vi "SMR_LabVIEW_V7.7.vi"() -> ()   [LabVIEW 2025]
uses:
  <vilib>/DAQmx/write.llb/DAQmx Write (Analog DBL 1Chan 1Samp).vi
  <vilib>/DAQmx/read.llb/DAQmx Read (Analog 1D DBL NChan 1Samp).vi
  <vilib>/DAQmx/read.llb/DAQmx Read (Analog 2D DBL NChan NSamp).vi
  <vilib>/Analysis/baseanly.llb/Mean (DBL).vi
  <vilib>/DAQmx/create/channels.llb/DAQmx Create Channel (AI-Temperature-Thermocouple).vi
  <vilib>/DAQmx/create/channels.llb/DAQmx Create Channel (AI-Voltage-Basic).vi
  <vilib>/DAQmx/create/channels.llb/DAQmx Create Channel (AO-Voltage-Basic).vi
  <vilib>/DAQmx/miscellaneous.llb/DAQmx Fill In Error Info.vi
  <vilib>/DAQmx/configure/timing.llb/DAQmx Timing (Sample Clock).vi
  <vilib>/addons/control/pid/pid.llb/PID (DBL).vi
  <vilib>/measure/maspectr.llb/FFT Power Spectrum and PSD for 1 Chan.vi
  <vilib>/measure/matone.llb/Extract Single Tone Information 1 Chan.vi
  <vilib>/addons/control/pid/NI_PID_pid.lvlib
  <vilib>/Analysis/NI_AALBase.lvlib
  <vilib>/ptbypt/NI_PtbyPt.lvlib
  <vilib>/measure/NI_MAPro.lvlib
panel:
  out "Main Loop Flow (GPM)":dbl
  out "FM Amplitude":dbl
  out "FM Frequency":dbl
  out "Spectrum":cluster{"f0":dbl, "df":dbl, "magnitude":dbl[]}(graph)
  out "Raw Signal":waveform(dbl)(graph)
  out "Smoothed HX Flow (GPM)":dbl
  out "Flow History":dbl(graph)
  out "HX Flow (GPM)":dbl
  out "Voltage Across Rod (V)":dbl format="%0.2f"
  out "Current Run Folder":path
  in  "Log Root Folder":path=path "C:/Users/LocalUser/Documents/GitHub/thermal-loop/resources/v0.1.1/data/001"
  out "Raw NI9201 \nVoltage Display":T1
  in  "Loop Period (ms)":dbl=1000.0
  in  "Stop":bool
  out "Auto Steady State Threshold (deg C/min)":dbl
  out "Max dT/dt (deg C/min)":dbl
  out "Temp Change Rate (deg C/min)":dbl
  out "5-Min Baseline Complete":bool
  out "Rate Window Ready":bool
  out "Steady State":bool
  in  "Voltage Limit (V)":dbl=10.0
  in  "Temperature Limit (C)":dbl=50.0
  in  "Pressure Limit (psi)":dbl=15.0
  out "Max Voltage":bool
  out "Max Temperature":bool
  out "Max Pressure":bool
  out "Heat Exchanger Pressure History":dbl(graph)
  out "Main Loop Pressure History":T2(graph)
  out "Overall Avg Pressure (psi)":dbl
  out "Heat Exchanger Pressure P6 (psi)":dbl
  out "Main Loop Avg Pressure (psi)":dbl
  out "Pressure Display":T3
  out "Overall Pressure History":T4(graph)
  out "Max Loop Pressure (psi)":dbl
  out "Heat Exchanger Temperature History":cluster{"Waveform":dbl, "Waveform":dbl}(graph)
  out "Main Loop Temeperature History":T5(graph)
  out "Heat Exchanger Avg Temp (deg C)":dbl
  out "Temperature Display":T6
  out "Overall Temperature History":T7(graph)
  out "Overall Avg Temp (deg C)":dbl
  out "Max Loop Temp (deg C)":dbl
  out "Final P-Valve Voltage (V)":dbl
  out "PID Trim Voltage (V)":dbl
  in  "PID Temp Setpoint (deg C)":dbl
  in  "Auto PID Enable":bool
  in  "Manual P-Valve Voltage (V)":dbl min=0.0 max=10.0
  out "Main Loop Avg Temp (deg C)":dbl
  # "Heat Exchanger Flow"
  # "Control/Troubleshoot"
  # "Steady State"
  # "Emergency Indicators"
  # "Pressure"
  # "Temperature"
  # "Proportional Valve Control"
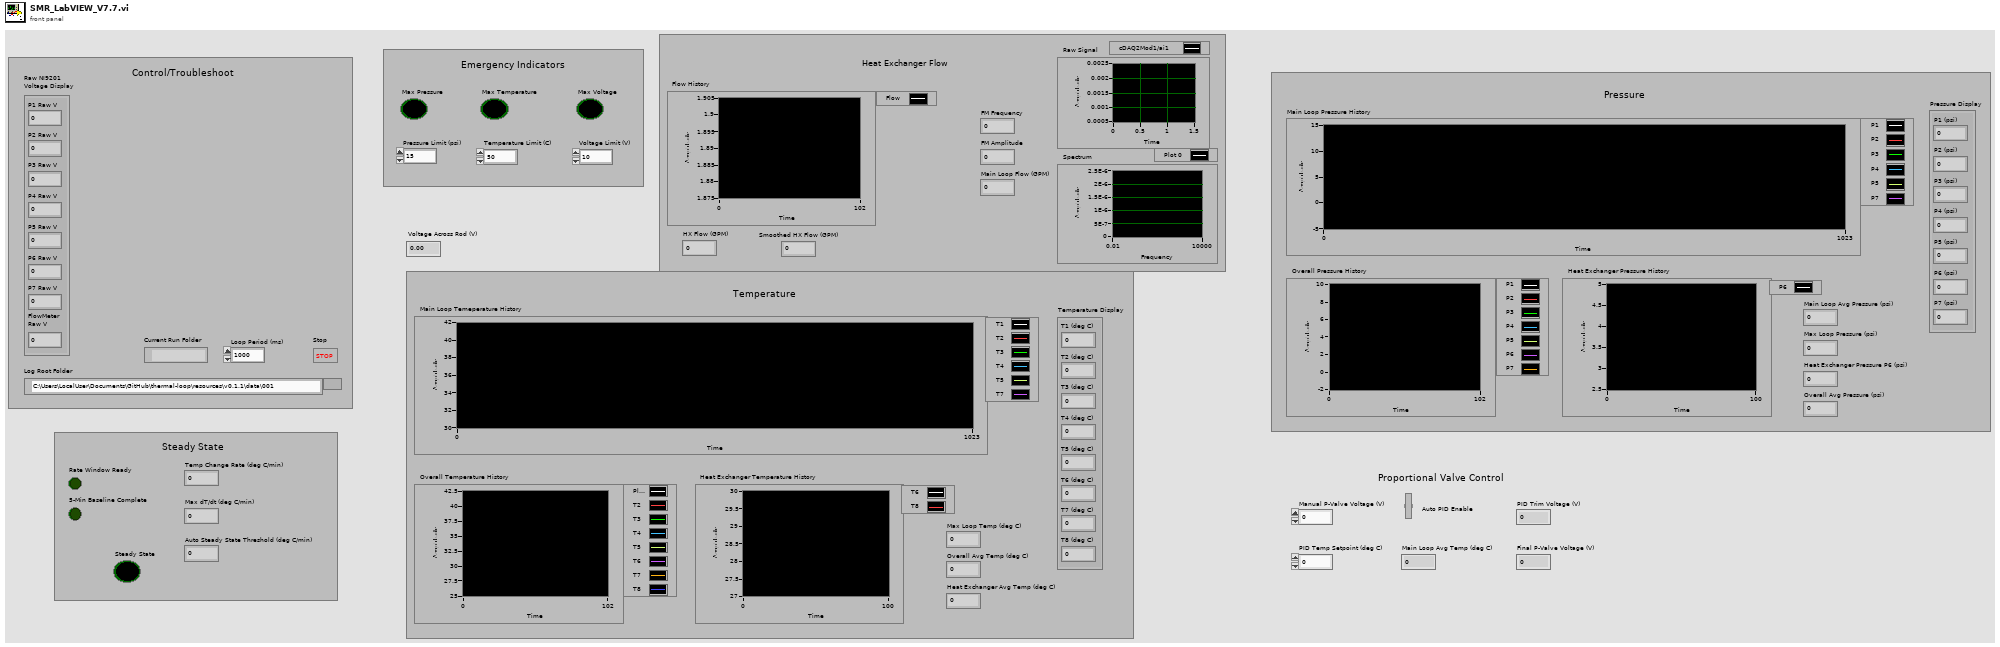
[diagram p1: front panel]
types:
  T1 = cluster{"P1 Raw V":dbl, "P2 Raw V":dbl, "P3 Raw V":dbl, "P4 Raw V":dbl, "P5 Raw V":dbl, "P6 Raw V":dbl, "P7 Raw V":dbl, "FlowMeter\nRaw V":dbl}
  T2 = cluster{"P1":dbl, "P2":dbl, "P3":dbl, "P4":dbl, "P5":dbl, "P7":dbl}
  T3 = cluster{"P1 (psi)":dbl, "P2 (psi)":dbl, "P3 (psi)":dbl, "P4 (psi)":dbl, "P5 (psi)":dbl, "P6 (psi)":dbl, "P7 (psi)":dbl}
  T4 = cluster{"P1":dbl, "P2":dbl, "P3":dbl, "P4":dbl, "P5":dbl, "P6":dbl, "P7":dbl}
  T5 = cluster{"Waveform":dbl, "Waveform":dbl, "Waveform":dbl, "Waveform":dbl, "Waveform":dbl, "Waveform":dbl}
  T6 = cluster{"T1 (deg C)":dbl, "T2 (deg C)":dbl, "T3 (deg C)":dbl, "T4 (deg C)":dbl, "T5 (deg C)":dbl, "T6 (deg C)":dbl, "T7 (deg C)":dbl, "T8 (deg C)":dbl}
  T7 = cluster{"Waveform":dbl, "Waveform":dbl, "Waveform":dbl, "Waveform":dbl, "Waveform":dbl, "Waveform":dbl, "Waveform":dbl, "Waveform":dbl}
  T8 = enum16{"open", "replace", "create", "open or create", "replace or create", "replace or create with confirmation"}
  T9 = cluster{"proportional gain (Kc)":dbl, "integral time (Ti, min)":dbl, "derivative time (Td, min)":dbl}
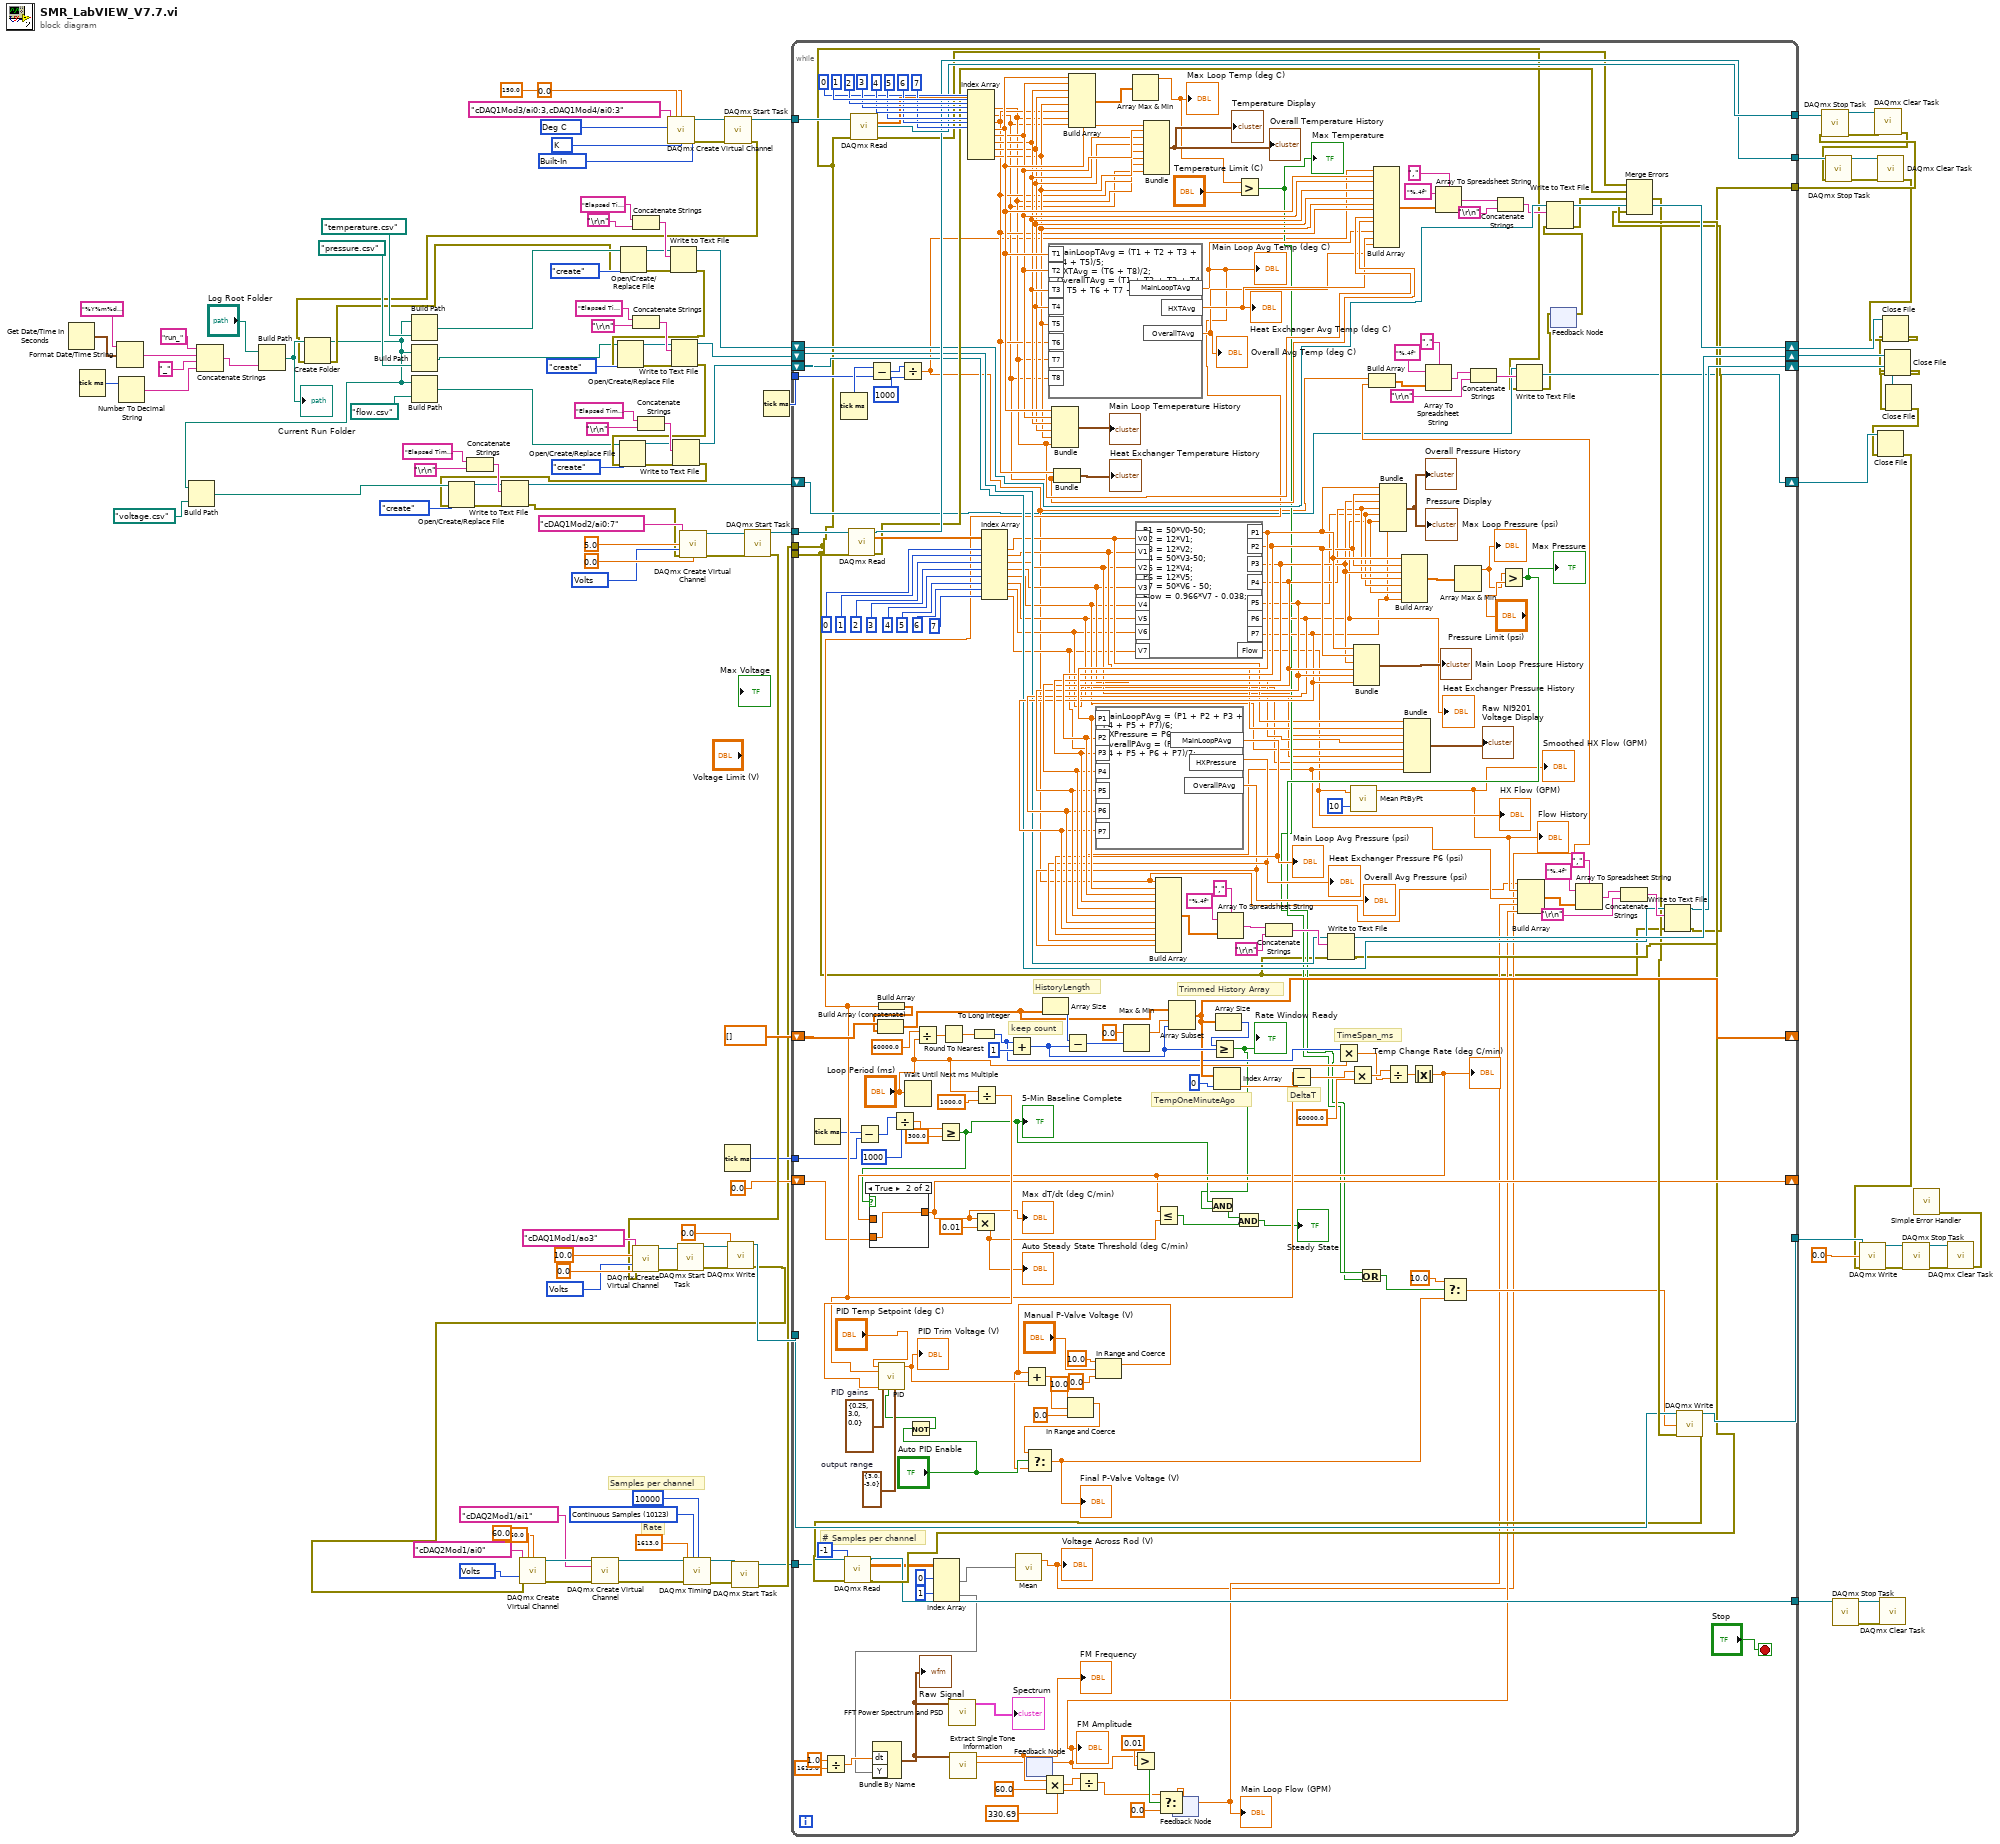
[diagram p0: block diagram]
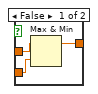
[diagram p2: hidden frame]
diagram:
  w30 = 10123 items=["Finite Samples"=10178, "Continuous Samples"=10123, "Hardware Timed Single Point"=12522] ("sample mode")
  w32 = 10348 items=["Volts"=10348, "From Custom Scale"=10065] ("units")
  w52 = 10348 items=["Volts"=10348, "From Custom Scale"=10065] ("units")
  w116 = 10200 items=["Built-In"=10200, "Constant Value"=10116, "Channel"=10113] ("cjc source")
  w117 = 10073 items=["J"=10072, "K"=10073, "N"=10077, "R"=10082, "S"=10085, "T"=10086, "B"=10047, "E"=10055] ("thermocouple type")
  w118 = 10143 items=["Deg C"=10143, "Deg F"=10144, "Kelvins"=10325, "Deg R"=10145, "From Custom Scale"=10065] ("units")
  w125 = 10348 items=["Volts"=10348, "From Custom Scale"=10065] ("units")
  # "Samples per channel"
  # "Rate"
  n1 = Get Date/Time In Seconds() -> (seconds since 1Jan1904=w74:timestamp)
  n2 = Tick Count (ms)() -> (millisecond timer value=w72:u32)
  n3 = Format Date/Time String(time format string (%c)="%Y%m%d_%H%M%S", seconds (now)=w74) -> (date/time string=w69:string)  [unwired: 1 in]
  n4 = Number To Decimal String(number=w72) -> (decimal integer string=w70:string)  [unwired: 1 in]
  n5 = Concatenate Strings("run_" ("string"), w69, "_" ("string"), w70) -> (w66:string)
  n6 = Build Path(base path="Log Root Folder", name or relative path=w66) -> (appended path=w65:path)
  "Current Run Folder" <- w65
  n7 = Concatenate Strings("Elapsed Time (s), Rod voltage (V)", "\r\n") -> (w14:string)
  n8 = Concatenate Strings("Elapsed Time (s),T1 (deg C),T2 (deg C),T3 (deg C),T4 (deg C),T5 (deg C),T6 (deg C),T7 (deg C),T8 (deg C),Main Loop Avg Temp (deg C),HX Avg Temp (deg C),Overall Avg Temp (deg C)", "\r\n") -> (w99:string)
  n9 = Concatenate Strings("Elapsed Time (s),P1 (psi),P2 (psi),P3 (psi),P4 (psi),P5 (psi),P6 (psi),P7 (psi),Main Loop Avg Pressure (psi),HX Pressure (psi),Overall Avg Pressure (psi)", "\r\n") -> (w97:string)
  n10 = Concatenate Strings("Elapsed Time (s),Heat Exchanger Flow (GPM),Flow Raw Voltage (V), Main Loop Flow (GPM), Flow Signal Amplitude (V)", "\r\n") -> (w93:string)
  n11 = call-poly <vilib>:"DAQmx Create Virtual Channel.vi"("maximum value"=150.0, "minimum value"=0.0, "physical channels"=tag "cDAQ1Mod3/ai0:3,cDAQ1Mod4/ai0:3", "cjc source"=w116, "units"=w118, "thermocouple type"=w117) -> ("task out"=w115:refnum<k21>, "error out"=w114:errorcluster)  [unwired: 8 in]
  n12 = Tick Count (ms)() -> (millisecond timer value=w37:u32)
  n13 = call <vilib>:"DAQmx Start Task.vi"("task/channels in"=w115, "error in"=w114) -> ("task out"=w113:refnum<k21>, "error out"=w58:errorcluster)  [unwired: 12 in]
  n14 = Create Folder(path (use dialog)=w65, error in=w58) -> (created path=w8:path, error out=w57:errorcluster)  [unwired: 1 in, 1 out]
  n15 = Build Path(base path=w8, name or relative path=path "voltage.csv") -> (appended path=w9:path)
  n16 = Build Path(base path=w8, name or relative path=path "temperature.csv") -> (appended path=w64:path)
  n17 = Build Path(base path=w8, name or relative path=path "pressure.csv") -> (appended path=w63:path)
  n18 = Build Path(base path=w8, name or relative path=path "flow.csv") -> (appended path=w62:path)
  n19 = Open/Create/Replace File(file path (use dialog)=w64, error in=w57, operation (0:open)=T8."create") -> (refnum out=w98:refnum<file>, error out=w82:errorcluster)  [unwired: 3 in, 1 out]
  n20 = Write to Text File(file (use dialog)=w98, text=w99, error in=w82) -> (refnum out=w89:refnum<file>, error out=w81:errorcluster)  [unwired: 1 in, 1 out]
  n21 = Open/Create/Replace File(file path (use dialog)=w63, error in=w81, operation (0:open)=T8."create") -> (refnum out=w96:refnum<file>, error out=w80:errorcluster)  [unwired: 3 in, 1 out]
  n22 = Write to Text File(file (use dialog)=w96, text=w97, error in=w80) -> (refnum out=w88:refnum<file>, error out=w79:errorcluster)  [unwired: 1 in, 1 out]
  n23 = Open/Create/Replace File(file path (use dialog)=w62, error in=w79, operation (0:open)=T8."create") -> (refnum out=w92:refnum<file>, error out=w78:errorcluster)  [unwired: 3 in, 1 out]
  n24 = Write to Text File(file (use dialog)=w92, text=w93, error in=w78) -> (refnum out=w87:refnum<file>, error out=w6:errorcluster)  [unwired: 1 in, 1 out]
  n25 = Open/Create/Replace File(file path (use dialog)=w9, error in=w6, operation (0:open)=T8."create") -> (refnum out=w13:refnum<file>, error out=w10:errorcluster)  [unwired: 3 in, 1 out]
  n26 = Write to Text File(file (use dialog)=w13, text=w14, error in=w10) -> (refnum out=w4:refnum<file>, error out=w5:errorcluster)  [unwired: 1 in, 1 out]
  n27 = call-poly <vilib>:"DAQmx Create Virtual Channel.vi"("maximum value"=5.0, "minimum value"=0.0, "physical channels"=tag "cDAQ1Mod2/ai0:7", "units"=w125, "error in"=w5) -> ("task out"=w124:refnum<k21>, "error out"=w123:errorcluster)  [unwired: 9 in]
  n28 = call <vilib>:"DAQmx Start Task.vi"("task/channels in"=w124, "error in"=w123) -> ("task out"=w122:refnum<k21>, "error out"=w45:errorcluster)  [unwired: 12 in]
  n29 = call-poly <vilib>:"DAQmx Create Virtual Channel.vi"("maximum value"=10.0, "minimum value"=0.0, "physical channels"=tag "cDAQ1Mod1/ao3", "units"=w52, "error in"=w45) -> ("task out"=w51:refnum<k21>, "error out"=w50:errorcluster)  [unwired: 9 in]
  n30 = call <vilib>:"DAQmx Start Task.vi"("task/channels in"=w51, "error in"=w50) -> ("task out"=w49:refnum<k21>, "error out"=w48:errorcluster)  [unwired: 12 in]
  n31 = call-poly <vilib>:"DAQmx Write.vi"("task/channels in"=w49, "data"=0.0, "error in"=w48) -> ("task out"=w46:refnum<k21>, "error out"=w24:errorcluster)  [unwired: 10 in, 1 out]
  n32 = call-poly <vilib>:"DAQmx Create Virtual Channel.vi"("maximum value"=60.0, "minimum value"=-60.0, "physical channels"=tag "cDAQ2Mod1/ai0", "units"=w32, "error in"=w24) -> ("task out"=w20:refnum<k21>, "error out"=w19:errorcluster)  [unwired: 9 in]
  n33 = call-poly <vilib>:"DAQmx Create Virtual Channel.vi"("task in"=w20, "physical channels"=tag "cDAQ2Mod1/ai1", "error in"=w19) -> ("task out"=w18:refnum<k21>, "error out"=w17:errorcluster)  [unwired: 11 in]
  n34 = call-poly <vilib>:"DAQmx Timing.vi"("task/channels in"=w18, "sample mode"=w30, "samples per channel"=10000, "rate"=1613.0, "error in"=w17) -> ("task out"=w28:refnum<k21>, "error out"=w27:errorcluster)  [unwired: 9 in]
  n35 = call <vilib>:"DAQmx Start Task.vi"("task/channels in"=w28, "error in"=w27) -> ("task out"=w22:refnum<k21>, "error out"=w23:errorcluster)  [unwired: 12 in]
  n36 = Tick Count (ms)() -> (millisecond timer value=w86:u32)
  n37 = while {
    tunnel: w122 -> [w330]
    tunnel: w113 -> [w313]
    tunnel: [w303] -> w112
    tunnel: [w131] -> _
    tunnel: [w302] -> w111
    tunnel: [w177] -> w110
    shift-right: [w279] -> w85
    shift-left: w89 -> [w280]
    shift-right: [w260] -> w84
    shift-left: w88 -> [w261]
    shift-right: [w252] -> w83
    shift-left: w87 -> [w253]
    tunnel: w86 -> [w298]
    shift-right: [w231] -> _
    shift-left: dbl[] [] -> [w244]
    tunnel: w46 -> [w212]
    tunnel: w23 -> [w131]
    tunnel: [w219] -> w43
    tunnel: w37 -> [w201]
    shift-right: [w194] -> _
    shift-left: 0.0 -> [w196]
    tunnel: w22 -> [w176]
    tunnel: [w175] -> w21
    shift-right: [w132] -> w3
    shift-left: w4 -> [w133]
    stop <- "Stop" stop-if-true
    w217 = cluster{"output high":dbl, "output low":dbl} {"output high"=3.0, "output low"=-3.0}  # output range
    w218 = T9 {"proportional gain (Kc)"=0.25, "integral time (Ti, min)"=3.0, "derivative time (Td, min)"=0.0}  # PID gains
    # "# Samples per channel"
    # "TimeSpan_ms"
    # "DeltaT"
    # "TempOneMinuteAgo"
    # "Trimmed History Array"
    # "HistoryLength"
    # "keep count"
    n38 = Tick Count (ms)() -> (millisecond timer value=w202:u32)
    n39 = Divide(x=1.0, y=1613.0) -> (x/y=w148:dbl)
    n40 = Tick Count (ms)() -> (millisecond timer value=w299:u32)
    n41 = call-poly <vilib>:"DAQmx Read.vi"("task/channels in"=w330, "error in"=w131) -> ("task out"=w302:refnum<k21>, "data"=w321:dbl[], "error out"=w300:errorcluster)  [unwired: 11 in]
    n42 = call-poly <vilib>:"DAQmx Read.vi"("task/channels in"=w313, "error in"=w131) -> ("task out"=w303:refnum<k21>, "data"=w304:dbl[], "error out"=w301:errorcluster)  [unwired: 11 in]
    n43 = Subtract(x=w202, y=w201) -> (x-y=w200:u32)
    n44 = Subtract(x=w299, y=w298) -> (x-y=w297:u32)
    n45 = Divide(x=w200, y=u32 1000) -> (x/y=w198:dbl)
    n46 = Divide(x=w297, y=u32 1000) -> (x/y=w136:dbl)
    n47 = Wait Until Next ms Multiple(millisecond multiple="Loop Period (ms)") -> ()  [unwired: 1 out]
    n48 = Not(x="Auto PID Enable") -> (.not. x?=w213:bool)
    n49 = Divide(x=60000.0, y="Loop Period (ms)") -> (x/y=w241:dbl)
    n50 = Greater Or Equal?(x=w198, y=300.0) -> (x >= y?=w191:bool)
    "5-Min Baseline Complete" <- w191
    n51 = Round To Nearest(number=w241) -> (nearest integer value=w240:dbl)
    n52 = Index Array(array=w304, index #1=0 ("index"), index #2=1 ("index"), index #3=2 ("index"), index #4=3 ("index"), index #5=4 ("index"), index #6=5 ("index"), index #7=6 ("index"), index #8=7 ("index")) -> (element #1=w289:dbl, element #2=w288:dbl, element #3=w290:dbl, element #4=w295:dbl, element #5=w294:dbl, element #6=w293:dbl, element #7=w292:dbl, element #8=w291:dbl)
    n53 = To Long Integer(number=w240) -> (32bit integer=w228:i32)
    n54 = Divide(x="Loop Period (ms)", y=1000.0) -> (x/y=w214:dbl)
    n55 = Index Array(array=w321, index #1=0 ("index"), index #2=1 ("index"), index #3=2 ("index"), index #4=3 ("index"), index #5=4 ("index"), index #6=5 ("index"), index #7=6 ("index"), index #8=7 ("index")) -> (element #1=w174:dbl, element #2=w173:dbl, element #3=w172:dbl, element #4=w171:dbl, element #5=w170:dbl, element #6=w169:dbl, element #7=w168:dbl, element #8=w167:dbl)
    n56 = Add(x=w228, y=1) -> (x+y=w233:i32)
    n57 = feedback #1() -> (w144:dbl)  [unwired: 1 in]
    "FM Amplitude" <- w144
    n58 = formula code="MainLoopTAvg = (T1 + T2 + T3 + T4 + T5)/5;\nHXTAvg = (T6 + T8)/2;\nOverallTAvg = (T1 + T2 + T3 + T4 + T5 + T6 + T7 + T8)/8;"("T1"=w295, "T2"=w294, "T3"=w293, "T4"=w292, "T5"=w291, "T6"=w290, "T7"=w289, "T8"=w288) -> ("MainLoopTAvg"=w204:dbl, "HXTAvg"=w287:dbl, "OverallTAvg"=w286:dbl)
    "Overall Avg Temp (deg C)" <- w286
    "Main Loop Avg Temp (deg C)" <- w204
    "Heat Exchanger Avg Temp (deg C)" <- w287
    n59 = Build Array(w204) -> (w243:dbl[])
    n60 = Build Array (concatenate)(w244, w243) -> (w235:dbl[])
    n61 = call-poly <vilib>:"PID.vi"("reinitialize? (F)"=w213, "output range"=w217, "dt (s)"=w214, "PID gains"=w218, "process variable"=w204, "setpoint"="PID Temp Setpoint (deg C)") -> ("output"=w211:dbl)  [unwired: 4 in, 1 out]
    "PID Trim Voltage (V)" <- w211
    n62 = Array Size(array=w235) -> (size(s)=w238:i32)
    n63 = Bundle("Waveform"=w295, "Waveform"=w294, "Waveform"=w293, "Waveform"=w292, "Waveform"=w291, "Waveform"=w289) -> (→"Main Loop Temeperature History":T5)  [unwired: 1 in]
    n64 = Bundle("Waveform"=w290, "Waveform"=w288) -> (→"Heat Exchanger Temperature History":cluster{"Waveform":dbl, "Waveform":dbl})  [unwired: 1 in]
    n65 = Subtract(x=w238, y=w233) -> (x-y=w236:i32)
    n66 = Build Array(w295, w294, w293, w292, w291, w290, w289, w288) -> (w331:dbl[])
    n67 = In Range and Coerce(upper limit=10.0, x="Manual P-Valve Voltage (V)", lower limit=0.0) -> (coerced(x)=w206:dbl)  [unwired: 1 out]
    n68 = Add(x=w206, y=w211) -> (x+y=w210:dbl)
    n69 = In Range and Coerce(upper limit=10.0, x=w210, lower limit=0.0) -> (coerced(x)=w205:dbl)  [unwired: 1 out]
    n70 = Select(t=w205, s="Auto PID Enable", f=w206) -> (s? t:f=w182:dbl)
    "Final P-Valve Voltage (V)" <- w182
    n71 = Max & Min(x=0.0, y=w236) -> (max(x,y)=w234:dbl)  [unwired: 1 out]
    n72 = Array Max & Min(array=w331) -> (max value=w246:dbl)  [unwired: 3 out]
    "Max Loop Temp (deg C)" <- w246
    n73 = Greater?(x=w144, y=0.01) -> (0:w152:bool)
    n74 = formula code="P1 = 50*V0-50;\nP2 = 12*V1;\nP3 = 12*V2;\nP4 = 50*V3-50;\nP5 = 12*V4;\nP6 = 12*V5; \nP7 = 50*V6 - 50;\nFlow = 0.966*V7 - 0.038;"("V0"=w174, "V1"=w173, "V2"=w172, "V3"=w171, "V4"=w170, "V5"=w169, "V6"=w168, "V7"=w167) -> ("P1"=w278:dbl, "P2"=w277:dbl, "P3"=w276:dbl, "P4"=w275:dbl, "P5"=w274:dbl, "P6"=w273:dbl, "P7"=w272:dbl, "Flow"=w166:dbl)
    "HX Flow (GPM)" <- w166
    "Heat Exchanger Pressure History" <- w273
    n75 = formula code="MainLoopPAvg = (P1 + P2 + P3 + P4 + P5 + P7)/6;\nHXPressure = P6;\nOverallPAvg = (P1 + P2 + P3 + P4 + P5 + P6 + P7)/7;"("P1"=w278, "P2"=w277, "P3"=w276, "P4"=w275, "P5"=w274, "P6"=w273, "P7"=w272) -> ("MainLoopPAvg"=w271:dbl, "HXPressure"=w270:dbl, "OverallPAvg"=w269:dbl)
    "Overall Avg Pressure (psi)" <- w269
    "Heat Exchanger Pressure P6 (psi)" <- w270
    "Main Loop Avg Pressure (psi)" <- w271
    n76 = Bundle("Waveform"=w295, "Waveform"=w294, "Waveform"=w293, "Waveform"=w292, "Waveform"=w291, "Waveform"=w290, "Waveform"=w289, "Waveform"=w288) -> (→"Overall Temperature History" →"Temperature Display":T7)  [unwired: 1 in]
    n77 = Build Array(w136, w278, w277, w276, w275, w274, w273, w272, w271, w270, w269) -> (w268:dbl[])
    n78 = Array Subset(array=w235, index=w234, length=w233) -> (w231:dbl[])
    n79 = feedback #2() -> (w142:dbl)  [unwired: 1 in]
    "Main Loop Flow (GPM)" <- w142
    n80 = Index Array(array=w231, index=0) -> (element=w229:dbl)
    n81 = Array Size(array=w231) -> (size(s)=w232:i32)
    n82 = Greater Or Equal?(x=w232, y=w233) -> (x >= y?=w190:bool)
    "Rate Window Ready" <- w190
    n83 = And(x=w191, y=w190) -> (x .and. y?=w189:bool)
    n84 = Array To Spreadsheet String(delimiter (Tab)=",", array=w268, 3:"%.4f" ("format string")) -> (spreadsheet string=w264:string)
    n85 = Greater?(x=w246, y="Temperature Limit (C)") -> (0:w185:bool)
    "Max Temperature" <- w185
    n86 = Concatenate Strings(w264, "\r\n") -> (w262:string)
    n87 = Subtract(x=w204, y=w229) -> (x-y=w227:dbl)
    n88 = Write to Text File(file (use dialog)=w261, text=w262, error in=w131) -> (refnum out=w260:refnum<file>, error out=w250:errorcluster)  [unwired: 1 in, 1 out]
    n89 = Multiply(x=w228, y="Loop Period (ms)") -> (x*y=w224:dbl)
    n90 = Multiply(x=w227, y=60000.0) -> (x*y=w225:dbl)
    n91 = call <vilib>:"Mean PtByPt.vi"("x"=w166, "sample length"=10) -> ("mean"=w164:dbl)  [unwired: 2 in, 1 out]
    "Flow History" <- w164
    "Smoothed HX Flow (GPM)" <- w164
    n92 = Bundle("P1"=w278, "P2"=w277, "P3"=w276, "P4"=w275, "P5"=w274, "P7"=w272) -> (→"Main Loop Pressure History":T2)  [unwired: 1 in]
    n93 = Build Array(w136, w295, w294, w293, w292, w291, w290, w289, w288, w204, w287, w286) -> (w285:dbl[])
    n94 = Bundle("P1"=w278, "P2"=w277, "P3"=w276, "P4"=w275, "P5"=w274, "P6"=w273, "P7"=w272) -> (→"Overall Pressure History" →"Pressure Display":T4)  [unwired: 1 in]
    n95 = Divide(x=w225, y=w224) -> (x/y=w223:dbl)
    n96 = Build Array(w278, w277, w276, w275, w274, w273, w272) -> (w320:dbl[])
    n97 = Bundle("Waveform"=w174, "Waveform"=w173, "Waveform"=w172, "Waveform"=w171, "Waveform"=w170, "Waveform"=w169, "Waveform"=w168, "Waveform"=w167) -> (→"Raw NI9201 \nVoltage Display":T7)  [unwired: 1 in]
    n98 = Absolute Value(x=w223) -> (abs(x)=w193:dbl)
    "Temp Change Rate (deg C/min)" <- w193
    n99 = case shown="True" w191 {
      tunnel: w196 -> [w335 w336]
      tunnel: w193 -> [w334 _]
      tunnel: [w333 w336] -> w194
      frame False {
        n100 = Max & Min(x=w334, y=w335) -> (max(x,y)=w333:dbl)  [unwired: 1 out]
      }
      frame True {
      }
    }
    "Max dT/dt (deg C/min)" <- w194
    n101 = Multiply(x=w194, y=0.01) -> (x*y=w192:dbl)
    "Auto Steady State Threshold (deg C/min)" <- w192
    n102 = Less Or Equal?(x=w193, y=w192) -> (x <= y?=w188:bool)
    n103 = And(x=w189, y=w188) -> (x .and. y?=→"Steady State":bool)
    n104 = Array To Spreadsheet String(delimiter (Tab)=",", array=w285, 3:"%.4f" ("format string")) -> (spreadsheet string=w282:string)
    n105 = Array Max & Min(array=w320) -> (max value=w247:dbl)  [unwired: 3 out]
    "Max Loop Pressure (psi)" <- w247
    n106 = Concatenate Strings(w282, "\r\n") -> (w265:string)
    n107 = Greater?(x=w247, y="Pressure Limit (psi)") -> (0:w186:bool)
    "Max Pressure" <- w186
    n108 = Or(x=w186, y=w185) -> (x .or. y?=w180:bool)
    n109 = Select(t=10.0, s=w180, f=w182) -> (s? t:f=w181:dbl)
    n110 = Build Array(w136, w164, w167, w142, w144) -> (w259:dbl[])
    n111 = feedback #3() -> (w129:errorcluster)  [unwired: 1 in]
    n112 = Write to Text File(file (use dialog)=w280, text=w265, error in=w129) -> (refnum out=w279:refnum<file>, error out=w251:errorcluster)  [unwired: 1 in, 1 out]
    n113 = Array To Spreadsheet String(delimiter (Tab)=",", array=w259, 3:"%.4f" ("format string")) -> (spreadsheet string=w255:string)
    n114 = Concatenate Strings(w255, "\r\n") -> (w254:string)
    n115 = Write to Text File(file (use dialog)=w253, text=w254, error in=w131) -> (refnum out=w252:refnum<file>, error out=w249:errorcluster)  [unwired: 1 in, 1 out]
    n116 = Merge Errors(w301, w300, w251, w250, w249) -> (w220:errorcluster)
    n117 = call-poly <vilib>:"DAQmx Write.vi"("task/channels in"=w212, "data"=w181, "error in"=w220) -> ("task out"=w219:refnum<k21>, "error out"=w178:errorcluster)  [unwired: 10 in, 1 out]
    n118 = call-poly <vilib>:"DAQmx Read.vi"("task/channels in"=w176, "number of samples per channel"=-1, "error in"=w178) -> ("task out"=w175:refnum<k21>, "data"=w163:dbl[][], "error out"=w177:errorcluster)  [unwired: 10 in]
    n119 = Index Array(array=w163, index (row) #1=0 ("index (row)"), index (row) #2=1 ("index (row)")) -> (element #1=w162:dbl[], element #2=w147:dbl[])  [unwired: 2 in]
    n120 = Bundle By Name("dt"=w148, "Y"=w147) -> (w146:waveform(dbl))  [unwired: 1 in]
    "Raw Signal" <- w146
    n121 = call-poly <vilib>:"FFT Power Spectrum and PSD.vi"("time signal"=w146) -> ("Power Spectrum / PSD"=→"Spectrum":cluster{"f0":dbl, "df":dbl, "magnitude":dbl[]})  [unwired: 7 in, 3 out]
    n122 = call-poly <vilib>:"Extract Single Tone Information.vi"("time signal in"=w146) -> ("detected amplitude"=w145:dbl, "detected frequency"=w158:dbl)  [unwired: 5 in, 4 out]
    "FM Frequency" <- w158
    n123 = call-poly <vilib>:"Mean.vi"("X"=w162) -> ("mean"=w137:dbl)  [unwired: 1 out]
    "Voltage Across Rod (V)" <- w137
    n124 = feedback-in #1(w145) -> ()
    n125 = Multiply(x=w158, y=60.0) -> (x*y=w156:dbl)
    n126 = Divide(x=w156, y=330.69) -> (x/y=w151:dbl)
    n127 = Select(t=w151, s=w152, f=0.0) -> (s? t:f=w143:dbl)
    n128 = feedback-in #2(w143) -> ()
    n129 = Build Array(w136, w137) -> (w135:dbl[])
    n130 = Array To Spreadsheet String(delimiter (Tab)=",", array=w135, 3:"%.4f" ("format string")) -> (spreadsheet string=w140:string)
    n131 = Concatenate Strings(w140, "\r\n") -> (w134:string)
    n132 = Write to Text File(file (use dialog)=w133, text=w134, error in=w131) -> (refnum out=w132:refnum<file>, error out=w130:errorcluster)  [unwired: 1 in, 1 out]
    n133 = feedback-in #3(w130) -> ()
  }
  n134 = call <vilib>:"DAQmx Stop Task.vi"("task/channels in"=w112, "error in"=w110) -> ("task out"=w109:refnum<k21>, "error out"=w107:errorcluster)  [unwired: 12 in]
  n135 = call <vilib>:"DAQmx Stop Task.vi"("task/channels in"=w21) -> ("task out"=w26:refnum<k21>, "error out"=w25:errorcluster)  [unwired: 13 in]
  n136 = call <vilib>:"DAQmx Clear Task.vi"("task in"=w109, "error in"=w107) -> ("error out"=w106:errorcluster)  [unwired: 13 in]
  n137 = call <vilib>:"DAQmx Stop Task.vi"("task/channels in"=w111, "error in"=w106) -> ("task out"=w108:refnum<k21>, "error out"=w105:errorcluster)  [unwired: 12 in]
  n138 = call <vilib>:"DAQmx Clear Task.vi"("task in"=w108, "error in"=w105) -> ("error out"=w77:errorcluster)  [unwired: 13 in]
  n139 = call <vilib>:"DAQmx Clear Task.vi"("task in"=w26, "error in"=w25) -> ()  [unwired: 13 in, 1 out]
  n140 = Close File(refnum=w85, error in=w77) -> (error out=w76:errorcluster)  [unwired: 1 out]
  n141 = Close File(refnum=w84, error in=w76) -> (error out=w75:errorcluster)  [unwired: 1 out]
  n142 = Close File(refnum=w83, error in=w75) -> (error out=w2:errorcluster)  [unwired: 1 out]
  n143 = Close File(refnum=w3, error in=w2) -> (error out=w1:errorcluster)  [unwired: 1 out]
  n144 = call-poly <vilib>:"DAQmx Write.vi"("task/channels in"=w43, "data"=0.0, "error in"=w1) -> ("task out"=w42:refnum<k21>, "error out"=w40:errorcluster)  [unwired: 10 in, 1 out]
  n145 = call <vilib>:"DAQmx Stop Task.vi"("task/channels in"=w42, "error in"=w40) -> ("task out"=w41:refnum<k21>, "error out"=w39:errorcluster)  [unwired: 12 in]
  n146 = call <vilib>:"DAQmx Clear Task.vi"("task in"=w41, "error in"=w39) -> ("error out"=w38:errorcluster)  [unwired: 13 in]
  n147 = call <vilib>:"Simple Error Handler.vi"("error in (no error)"=w38) -> ()  [unwired: 4 in, 5 out]
